vi "Insert Element at Start.vi"(8 "error in (no error)":errorcluster, 9 "element":variant, 10 "Name":string, 11 "Variant (Cluster) in":variant) -> (0 "error out":errorcluster, 3 "Variant (Cluster) out":variant)   [LabVIEW 2017, in "Variant Data Manipulation.lvlib"]
uses:
  Variant Data Manipulation.lvlib
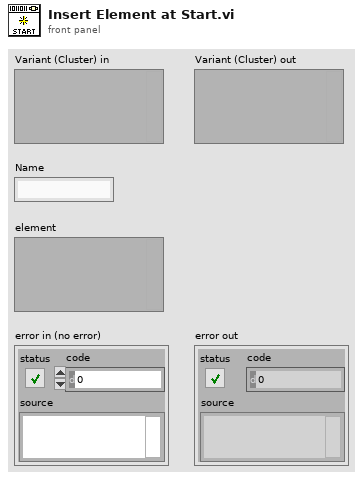
[diagram p1: front panel]
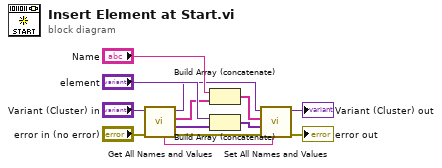
[diagram p0: block diagram]
diagram:
  n1 = call "Get All Names and Values.vi"("error in"="error in (no error)", "Cluster in"="Variant (Cluster) in") -> ("error out"=w11:errorcluster, "Values"=w12:variant[], "Element Names"=w5:string[], "Cluster out"=w1:variant, "Cluster Name"=w2:string)  [unwired: 5 in]
  n2 = Build Array (concatenate)("Name", w5) -> (w3:string[])
  n3 = Build Array (concatenate)("element", w12) -> (w8:variant[])
  n4 = call "Set All Names and Values.vi"("Cluster Name"=w2, "error in"=w11, "values"=w8, "Element Names"=w3, "Cluster in"=w1) -> ("error out"=→"error out":errorcluster, "Cluster out"=→"Variant (Cluster) out":variant)  [unwired: 5 in]
